vi "Set Write Decimation.vi"(8 "error in (no error)":errorcluster, 10 "Write Decimation":u32, 11 "Custom Device reference in":refnum<k24>) -> (0 "error out":errorcluster, 3 "Custom Device reference out":refnum<k24>)   [LabVIEW 2013, in "J1939 System Definition API Support.lvlib"]
uses:
  J1939 System Definition API Support.lvlib
  NationalInstruments.VeriStand.SystemDefinitionAPI
  Shared/SubVIs/Constants.vi
  <vilib>/NI Veristand/Custom Device Tools/Custom Device Utility Library/NI VeriStand - Search for Item by GUID.vi
  <vilib>/NI Veristand/Custom Device API/Set Item Property (U32).vi
  <vilib>/NI Veristand/Custom Device Tools/Custom Device Utility Library/Custom Device Utility Library.lvlib
  Shared/J1939 Addon Shared.lvlib
  <vilib>/NI Veristand/Custom Device API/Custom Device API.lvlib
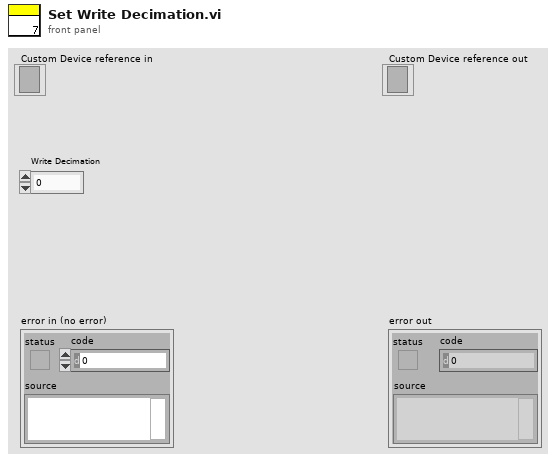
[diagram p1: front panel]
types:
  T1 = typedef "Custom Device API.lvlib/Custom Device Item Ref.ctl" = u64
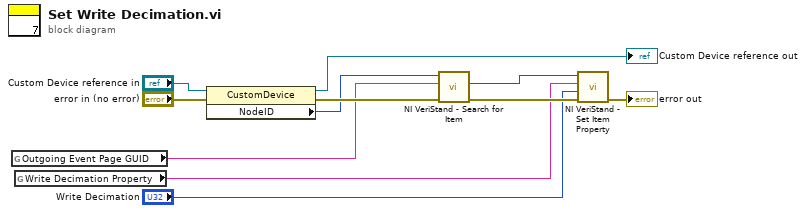
[diagram p0: block diagram]
diagram:
  n1 = global read "Constants.vi" "Outgoing Event Page GUID"() -> (w6:string)
  n2 = global read "Constants.vi" "Write Decimation Property"() -> (w3:string)
  n3 = property class="CustomDevice"(reference="Custom Device reference in", error in="error in (no error)") -> (reference out=→"Custom Device reference out":refnum<k24>, error out=w8:errorcluster, "NodeID"=w7:u64)
  n4 = call-poly <vilib>:"NI VeriStand - Search for Item.vi"("error in"=w8, "Item GUID"=w6, "Section Ref in"=w7) -> ("error out"=w4:errorcluster, "Item Ref"=w5:T1)  [unwired: 5 in, 2 out]
  n5 = call-poly <vilib>:"NI VeriStand - Set Item Property.vi"("error in (no error)"=w4, "Value"="Write Decimation", "Property Name"=w3, "Item Ref in"=w5) -> ("error out"=→"error out":errorcluster)  [unwired: 5 in, 2 out]
